vi "CLD 11Unbundle data SubVI.vi"(8 "error in (no error)":errorcluster, 10 "Current State Number":i32, 11 "[Data In]":T1[](array[typedef])) -> (0 "error out":errorcluster, 1 "State 3":bool, 2 "State 2":bool, 3 "[Data Out]":T1[](array[typedef]), 4 "Next Dwell TIme":dbl, 5 "State 1":bool, 6 "Dwell Time":dbl)   [LabVIEW 2018]
doc: "CLD 11. Data unbundle utility. Copied from CLD 10 solution."
uses:
  CLD 11 CSV file data structure.ctl
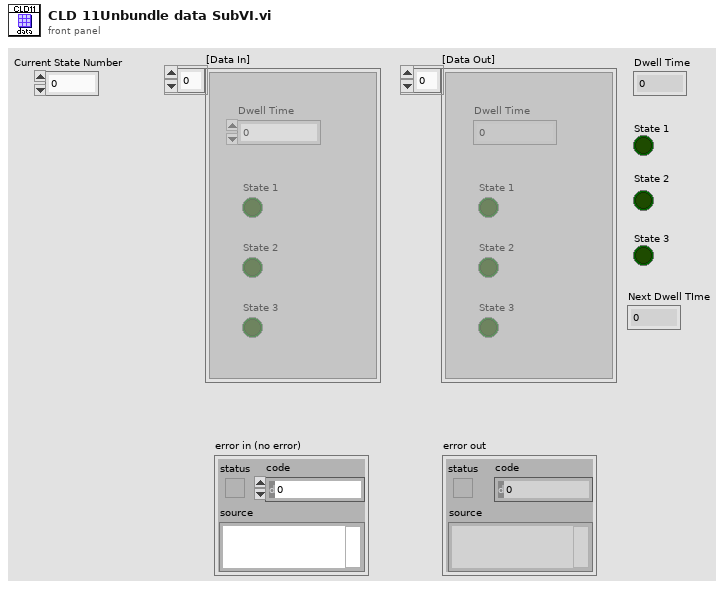
[diagram p1: front panel]
types:
  T1 = typedef "CLD 11 CSV file data structure.ctl" = cluster{"Dwell Time":i32, "State 1":bool, "State 2":bool, "State 3":bool}
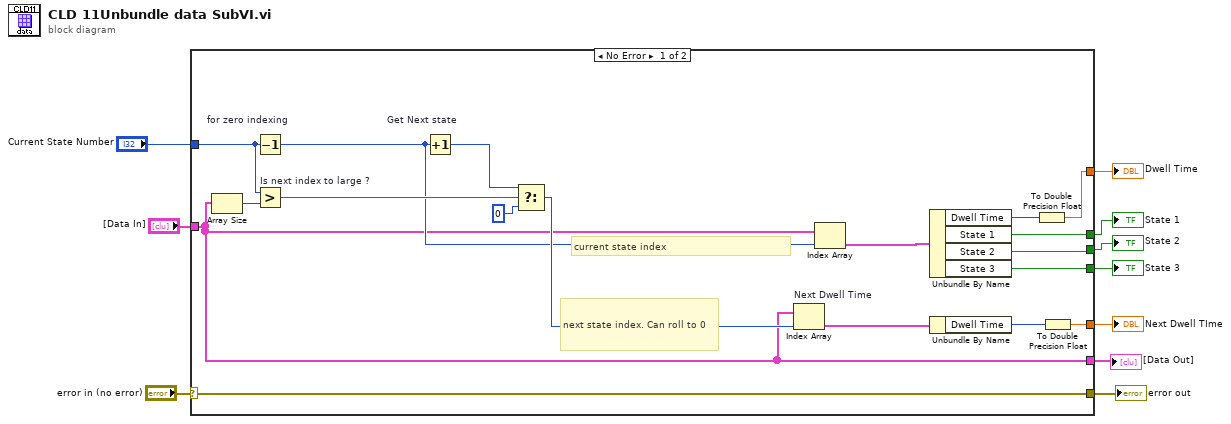
[diagram p0: block diagram]
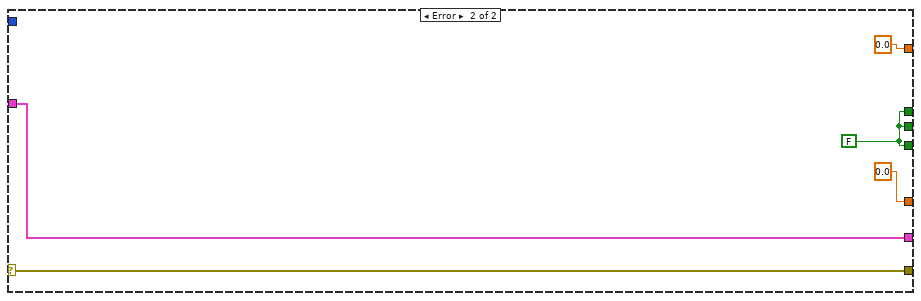
[diagram p2: hidden frame]
diagram:
  n1 = case shown="No Error" "error in (no error)" {
    selector: "error in (no error)" -> [w16 w31]
    tunnel: [w26 0.0] -> w10
    tunnel: "[Data In]" -> [w12 w29]
    tunnel: [w18 0.0] -> w8
    tunnel: [w16 w31] -> w6
    tunnel: [w15 w30] -> w5
    tunnel: [w14 w30] -> w4
    tunnel: [w13 w30] -> w3
    tunnel: [w12 w29] -> w2
    tunnel: "Current State Number" -> [w11 _]
    frame No Error {
      # "next state index. Can roll to 0"
      # "current state index"
      n2 = Array Size(array=w12) -> (size(s)=w22:i32)
      n3 = Decrement "for zero indexing"(x=w11) -> (x-1=w17:i32)
      n4 = Greater? "Is next index to large ?"(x=w11, y=w22) -> (0:w25:bool)
      n5 = Increment "Get Next state"(x=w17) -> (x+1=w21:i32)
      n6 = Select(t=w21, s=w25, f=0) -> (s? t:f=w23:i32)
      n7 = Index Array "Next Dwell Time"(array=w12, index=w23) -> (element=w20:T1)
      n8 = Index Array(array=w12, index=w17) -> (element=w28:T1)
      n9 = Unbundle By Name(w28) -> ("Dwell Time"=w27:i32, "State 1"=w15:bool, "State 2"=w14:bool, "State 3"=w13:bool)
      n10 = Unbundle By Name(w20) -> ("Dwell Time"=w19:i32)
      n11 = To Double Precision Float(number=w27) -> (double precision float=w26:dbl)
      n12 = To Double Precision Float(number=w19) -> (double precision float=w18:dbl)
    }
    frame Error {
      w30 = FALSE ("State 1")
    }
  }
  "Dwell Time" <- w10
  "Next Dwell TIme" <- w8
  "error out" <- w6
  "State 1" <- w5
  "State 2" <- w4
  "State 3" <- w3
  "[Data Out]" <- w2
